vi "Day 4.vi"() -> ()   [LabVIEW 2020]
uses:
  Typedefs/Passport.ctl
  Typedefs/ecl.ctl
panel:
  out "Array 3":T1(array[cluster])
  out "Failures Only":string[](array[string])
  out "Array 2":bool[](array[boolean])
  out "sum":i16
  out "Array":T2[](array[typedef])
  out "output array":string[](array[string])
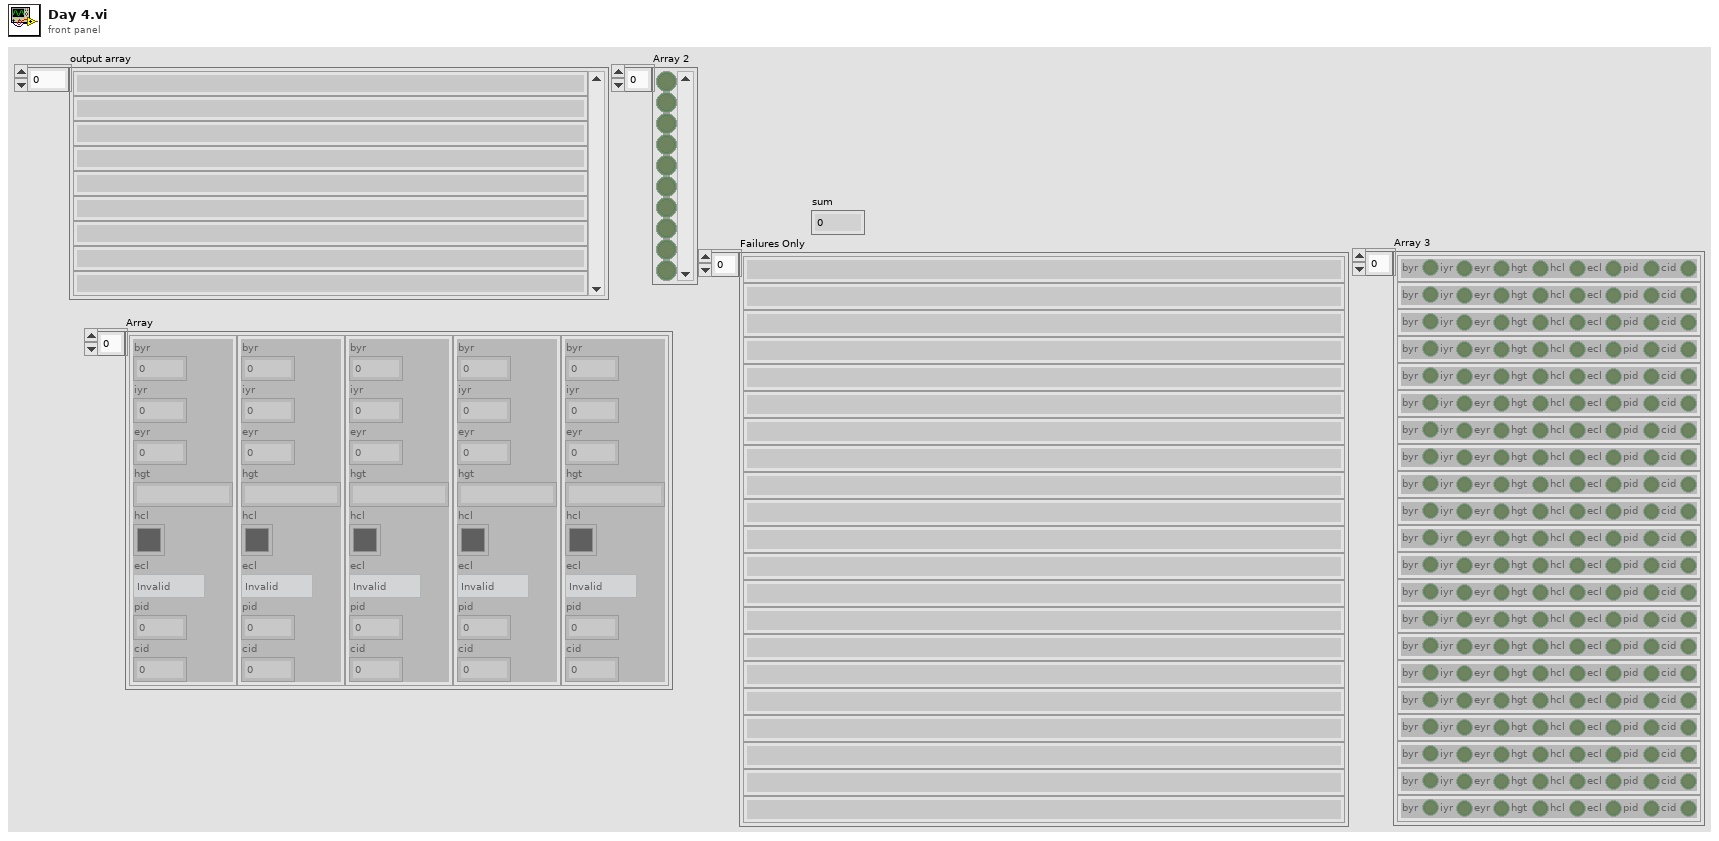
[diagram p1: front panel]
types:
  T1 = cluster{"byr":bool, "iyr":bool, "eyr":bool, "hgt":bool, "hcl":bool, "ecl":bool, "pid":bool, "cid":bool}[]
  T2 = typedef "Passport.ctl" = cluster{"byr":i32, "iyr":i32, "eyr":i32, "hgt":string, "hcl":u32, "ecl":T3, "pid":i32, "cid":i32}
  T3 = typedef "ecl.ctl" = enum16{"Invalid", "amb", "blu", "brn", "gry", "grn", "hzl", "oth"}
  T4 = cluster{"byr":bool, "iyr":bool, "eyr":bool, "hgt":bool, "hcl":bool, "ecl":bool, "pid":bool, "cid":bool}
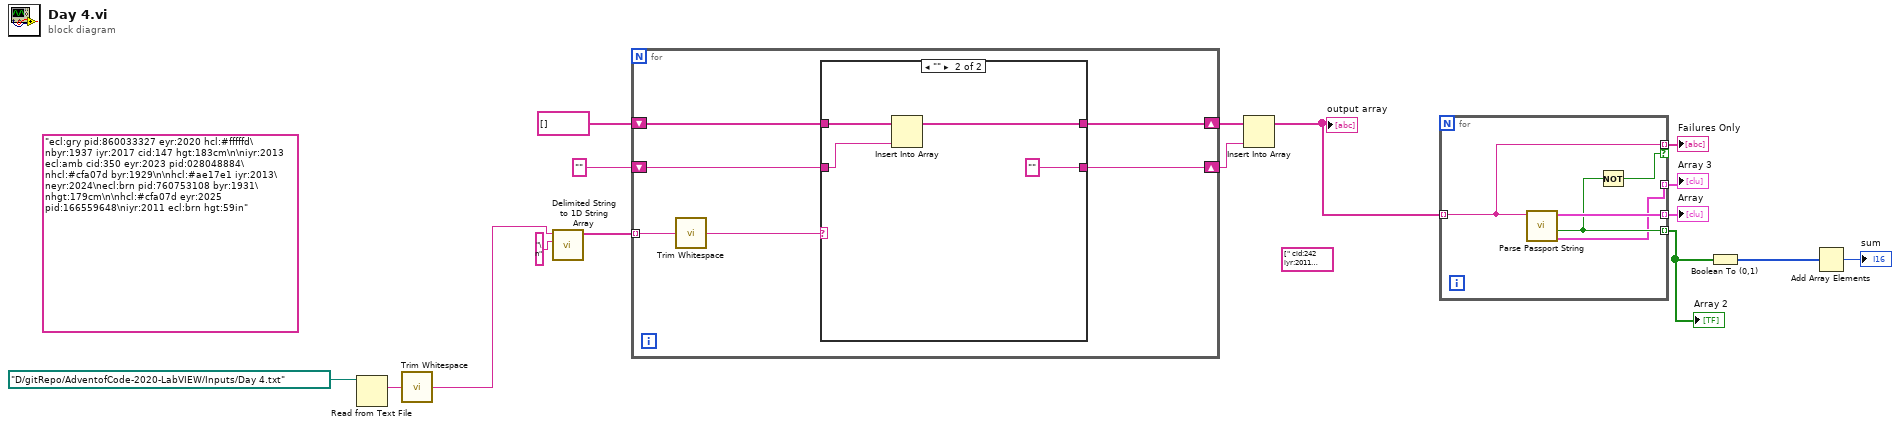
[diagram p0: block diagram]
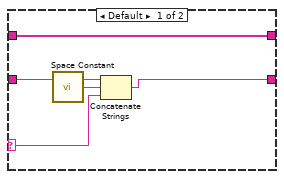
[diagram p2: hidden frame]
diagram:
  (unwired) string[] [" cid:242 iyr:2011 pid:953198122 eyr:2029 ecl:blu hcl:#888785", " hcl:#fffffd hgt:152cm byr:1996 ecl:gry eyr:2024", " pid:328737320 iyr:2017 hcl:#fffffd hgt:178 ecl:#35fad5 byr:1959", " iyr:2010 byr:1943 eyr:2028 hgt:178cm hcl:#888785 pid:572750267", " hgt:182cm ecl:blu eyr:2028 iyr:2011 hcl:#a97842 pid:758494126", " iyr:2023 hgt:174cm hcl:cafc2f ecl:utc cid:299 eyr:2026 pid:57963956", " ecl:amb hgt:70 iyr:2018 pid:241872490 byr:1962 eyr:2024 hcl:c5f0c3", " pid:994754974 eyr:2029 iyr:2017 cid:137 byr:1966 hcl:#733820 ecl:blu", " ecl:utc pid:937481632 hgt:190 eyr:2025 iyr:2027 byr:1949 cid:84 hcl:d3f4f5", " byr:2010 hgt:181cm iyr:2020 eyr:2040 pid:785862801 ecl:#f84ccd", " cid:314 hgt:180cm ecl:amb hcl:#602927 byr:2027 iyr:1958 eyr:2020 pid:#b2b732", " eyr:2030 pid:783631610 hgt:74 byr:2014 hcl:z iyr:2003 ecl:grt", " ecl:#d4d852 iyr:2029 hcl:z hgt:185in eyr:2034 pid:#526166", " iyr:1946 eyr:1957 byr:1941 pid:632690435 ecl:oth hcl:18a37c hgt:59cm", " iyr:2013 eyr:2026 pid:002380966 cid:95 hcl:#623a2f byr:1965 ecl:oth", " ecl:#5d8b3b hgt:156cm eyr:2029 pid:#3df0cc byr:1967 cid:118 hcl:e23f0f", " byr:1966 hgt:158cm eyr:2029 hcl:#602927 iyr:2013 pid:963663665", " hcl:#fffffd ecl:gry cid:93 pid:731904973 byr:1939 eyr:2029 iyr:2016", " pid:96716037 iyr:1938 eyr:2032 hgt:192 ecl:gmt byr:2029 hcl:02edc5", " byr:1958 iyr:2011 eyr:2029 ecl:gry pid:526931024 hcl:z hgt:59cm", " pid:1134356373 iyr:2019 ecl:grn hcl:#ceb3a1 byr:1950 hgt:154in", " hgt:157cm ecl:zzz byr:1976 pid:5047305958 iyr:2013 hcl:#341e13", " iyr:2029 ecl:#559ffe hcl:z cid:156 byr:2003 hgt:178 pid:93994500", " iyr:2026 hcl:#eda7f3 ecl:amb byr:1921 eyr:2021 pid:153cm", " pid:555636800 eyr:2020 hgt:182cm iyr:2019 byr:1948 cid:325 hcl:#733820", " eyr:1973 iyr:2024 hcl:z byr:2028 ecl:dne cid:169 pid:43596015 hgt:170in", " iyr:2013 hcl:z hgt:73cm byr:2014 pid:192cm ecl:#1627a7", " pid:816749378 hgt:178cm hcl:#733820 eyr:2029 byr:1993", " hcl:0cacc5 byr:1944 iyr:2028 eyr:2024 hgt:163in pid:74169361 ecl:dne", " hcl:#ceb3a1 ecl:grn eyr:2027 pid:481186415 hgt:176cm cid:325 byr:1986", " ecl:brn cid:323 hgt:167 byr:1993 iyr:1953 hcl:z eyr:2023 pid:161542750", " ecl:#895336 eyr:2033 hgt:67cm cid:254 iyr:1967 hcl:z byr:1954", " ecl:utc iyr:2014 hgt:183in byr:2007 eyr:2026 hcl:#cfa07d cid:334", " ecl:gry hcl:#b6652a pid:250420128 eyr:2024 byr:1939 hgt:170cm", " hgt:129 byr:2016 hcl:6734a1 ecl:#915282 iyr:1949 cid:130 pid:677408864 eyr:2030", " ecl:grn iyr:2019 pid:775867641 hcl:#bf1e29 byr:1920 hgt:163cm", " iyr:2019 ecl:#19fef5 pid:2080468234 eyr:2008 hgt:72 hcl:e14dfe byr:1980 cid:272", " byr:2025 cid:163 iyr:2020 pid:758946748 hgt:161cm ecl:amb eyr:2023 hcl:026d4d", " eyr:2023 hcl:z iyr:2019 byr:2013 ecl:#b42611 pid:164cm hgt:60cm", " cid:168 pid:#8556c9 hcl:413944 eyr:2036 byr:2013 iyr:2012 ecl:#66dc1c hgt:59cm", " eyr:1984 byr:2017 pid:#cbc84e hcl:z cid:189 iyr:2021 ecl:blu hgt:152cm", " hgt:172 byr:2008 eyr:2030 iyr:1959 ecl:oth hcl:#a8ebbb", " iyr:2013 hcl:#8f97b1 hgt:182cm ecl:grn cid:89 eyr:2029 byr:1974", " hcl:z pid:85905429 byr:1923 cid:260 eyr:2031 ecl:gry iyr:2022 hgt:180cm", " ecl:oth pid:087762106 hgt:190cm byr:1974 cid:171 hcl:#c63f21 eyr:2020", " hgt:170cm eyr:2021 cid:219 hcl:#a97842 pid:040224991 byr:1950 iyr:2018", " byr:2029 eyr:2036 cid:309 iyr:2016 hgt:167cm hcl:#fffffd ecl:#1ab23b", " eyr:2029 pid:669044398 hgt:161cm hcl:#cfa07d ecl:gry iyr:2018", " iyr:2013 eyr:2027 cid:223 pid:145547438 hcl:#6e6f47 hgt:165cm ecl:amb", " eyr:2026 hcl:z byr:2018 pid:7809314464 iyr:2012 hgt:158cm ecl:hzl", " cid:291 hgt:168 ecl:#7734de iyr:2021 hcl:5b4ef1 pid:3381158334 eyr:1956 byr:2003", " pid:68300657 byr:1988 hgt:181cm ecl:hzl iyr:1951 hcl:e18469 eyr:2013", " pid:157572693 hgt:185cm hcl:#065fe8 ecl:gry eyr:2027 iyr:2014", " eyr:2029 hgt:164cm hcl:z ecl:grn cid:270 iyr:2019 byr:1993 pid:338068138", " iyr:2019 eyr:2024 hgt:174cm pid:855792798 byr:1920 hcl:#cfa07d", " eyr:2020 hgt:74in iyr:2013 ecl:amb byr:1920 hcl:3f6214 pid:957164804", " byr:2021 hcl:ca4bcf hgt:88 iyr:2017 ecl:gmt pid:181cm eyr:2032", " iyr:2002 cid:139 byr:1982 hcl:#c0946f pid:#62721b hgt:159in eyr:1966 ecl:brn", " eyr:2036 ecl:oth byr:2026 hgt:96 pid:137651094 hcl:z", " pid:373485985 iyr:2030 ecl:gry byr:2011 hgt:65cm hcl:#733820", " pid:#fd3377 ecl:#618bce hcl:#ceb3a1 iyr:1944 hgt:182cm cid:57 byr:2022 eyr:1995", " pid:4790730010 hgt:192cm cid:222 byr:2022 hcl:4798e7 ecl:#5126d5 iyr:1954 eyr:2040", " iyr:1979 hcl:e09b9c byr:2016 hgt:121 eyr:1962 pid:#fb14be cid:265 ecl:lzr", " ecl:#fe1b74 iyr:1926 hgt:70cm pid:70807766 hcl:556dca byr:2030 eyr:2032", " eyr:2039 byr:2025 pid:247367429 hcl:z iyr:2013 ecl:amb cid:118", " eyr:2027 hcl:z ecl:utc cid:274 hgt:175in iyr:2016 byr:1977 pid:478855994", " ecl:utc byr:2026 iyr:1999 eyr:1937 hgt:66cm hcl:z pid:2247643960", " ecl:xry pid:346719476 iyr:1999 eyr:2020 hgt:154cm hcl:z byr:2027", " iyr:2010 hcl:#efcc98 pid:351846405 eyr:2024 hgt:150cm byr:1941", " byr:1994 eyr:2028 ecl:gry hcl:#888785 iyr:2010 hgt:165cm cid:183", " eyr:2031 hcl:6804ef ecl:amb byr:2024 hgt:157cm iyr:1938 pid:#0418fb", " pid:381452527 eyr:2027 hcl:#efcc98 ecl:brn byr:1956 hgt:63in", " byr:1968 pid:875469219 hcl:#efcc98 hgt:176cm cid:141 iyr:2017", " byr:1947 hcl:z cid:188 eyr:2038 pid:177cm iyr:2011 hgt:166cm ecl:#c1376b", " ecl:hzl hgt:170cm cid:307 eyr:2022 byr:1971 hcl:#b6652a pid:047040501", " hgt:126 ecl:zzz byr:2019 pid:170207910 eyr:2035 hcl:23df48 iyr:1932", " hgt:152cm cid:270 eyr:2036 ecl:#408f6e iyr:1952 pid:5808880830 byr:2022 hcl:0b1ba6", " hgt:67cm eyr:2028 pid:816355657 iyr:2019 byr:2008 hcl:z ecl:#5b4f31", " byr:1955 hgt:71in iyr:2018 pid:320019385 hcl:#6b5442 cid:324 eyr:2027", " pid:957860464 hcl:#602927 iyr:2011 byr:2026 cid:261 eyr:2006", " pid:#1742ae ecl:#a61090 iyr:2028 hcl:717dd0 hgt:139 cid:183 eyr:2035", " ecl:#4004e3 cid:278 iyr:1950 pid:745107377 byr:2007 eyr:2036 hcl:8447eb hgt:74cm", " hgt:187cm iyr:1921 ecl:#1c7d96 eyr:1987 byr:2028 pid:#28e5a1 cid:144 hcl:9fc25d", " pid:860410143 ecl:dne eyr:2031 cid:206 hgt:187in byr:1927 hcl:8c2149 iyr:2012", " iyr:2010 byr:1963 cid:139 pid:160019759 eyr:2030 hgt:172cm hcl:#602927", " byr:2023 ecl:brn cid:101 eyr:2016 pid:190078757 hgt:188in", " byr:2011 hcl:z ecl:gry pid:408316491 hgt:64cm iyr:2017 eyr:1968", " ecl:oth hcl:#6b5442 pid:623099801 hgt:163cm byr:1928", " pid:165230004 ecl:grn byr:1935 hcl:#c0946f iyr:2012 hgt:185cm", " ecl:#f3d8ba hgt:182cm eyr:2020 byr:2007 hcl:z iyr:2014 pid:6141297559", " pid:867747198 hcl:#efcc98 eyr:2030 byr:1989 hgt:181cm", " eyr:2034 hcl:#623a2f byr:1958 pid:60553207 ecl:#76b538 hgt:59 cid:75", " ecl:grn eyr:2036 iyr:1951 byr:2029 hcl:z hgt:177in pid:135470038", " byr:2014 pid:25253929 hcl:z ecl:#f3fb41 eyr:2025 cid:255 iyr:1998 hgt:155cm", " ecl:gry pid:919070381 hcl:#efcc98 iyr:2019 eyr:2021 byr:1995", " ecl:gry byr:1963 iyr:2016 hgt:188cm pid:024539026 eyr:2022", " iyr:2011 hcl:#888785 eyr:2030 ecl:gry byr:1920", " pid:#0468a7 hcl:851fe0 eyr:2036 hgt:60cm byr:2030 iyr:1995 ecl:utc", " cid:185 ecl:#5f6f53 pid:#20f317 byr:2024 eyr:1988 hcl:z iyr:2023 hgt:158in", " pid:782547454 hcl:z ecl:#b0805f iyr:2013 eyr:2023 hgt:159cm byr:1935 cid:230", " pid:298008321 hcl:231e1b hgt:166cm ecl:oth iyr:2026 eyr:2020", " pid:230201309 iyr:2010 eyr:2025 hcl:#6b5442 cid:238 ecl:grn hgt:174cm", " iyr:2020 byr:1938 pid:927067439 eyr:2027 hgt:173cm hcl:306963 ecl:xry", " byr:1991 iyr:2021 hgt:175cm hcl:68b4f3 ecl:utc pid:037777327 eyr:2026", " byr:1938 eyr:2021 pid:575395401 cid:234 hcl:#866857 ecl:hzl hgt:176cm", " hcl:#ceb3a1 ecl:hzl eyr:2035 iyr:2014 byr:2019", " eyr:1936 ecl:blu hgt:153cm hcl:98d3f0 pid:7296832671 byr:1931 iyr:1962", " pid:203025149 eyr:2029 iyr:2010 cid:124 byr:1999 ecl:blu", " iyr:2011 eyr:2028 pid:#7e0612 byr:1924 hcl:#7d3b0c ecl:oth hgt:82", " pid:#49ea2c eyr:2029 hcl:#6b5442 iyr:1931 hgt:62cm ecl:brn byr:2012", " eyr:2038 hcl:8d1f49 ecl:#6d4ea1 pid:0853660207 byr:2020 hgt:71cm", " byr:1921 hcl:#c0946f ecl:blu iyr:2019 eyr:2024 pid:643387204", " byr:2004 iyr:2022 pid:157cm eyr:2035 ecl:#eafe47 hgt:129 hcl:z", " byr:1930 hcl:5bdf31 pid:#b21f8a hgt:164cm cid:134 iyr:2023 ecl:lzr", " hcl:2a1c4f iyr:2011 hgt:192cm eyr:2028 byr:2029 cid:270 ecl:dne pid:7995627426", " eyr:2022 iyr:2018 byr:1972 cid:290 hgt:170cm ecl:grn pid:127269636", " pid:571765355 byr:2021 hcl:z eyr:1921 cid:106 iyr:1978 ecl:#1162c5 hgt:184in", " ecl:hzl pid:484466493 hgt:176cm iyr:2016 byr:1983 hcl:#ceb3a1", " ecl:brn hcl:352cf1 cid:149 hgt:184cm byr:2011 eyr:2031 pid:21942403 iyr:2028", " ecl:gry hcl:#18171d iyr:2015 hgt:185cm eyr:2023 byr:1950", " iyr:2003 eyr:2020 cid:99 byr:2027 hcl:2c10a6 hgt:74cm ecl:brn", " pid:151cm hcl:46a5fd eyr:2031 iyr:2014 byr:2005 ecl:xry hgt:176cm", " byr:2011 ecl:oth pid:821123244 iyr:2022 hcl:839b47 eyr:2039 hgt:150in", " iyr:2018 hgt:164cm hcl:#650d28 byr:1973 cid:108 pid:#b0df80 ecl:blu eyr:2020", " hcl:z pid:315901778 iyr:2013 byr:1999 ecl:#49f691 eyr:2026 hgt:179cm", " pid:163cm hgt:189cm iyr:1997 hcl:03db25 eyr:1970 byr:2016 ecl:#6c59eb", " pid:766719295 iyr:2017 hgt:168cm hcl:z ecl:grt eyr:2022 byr:2010", " hgt:173cm pid:247156751 cid:109 eyr:2022 iyr:2012 ecl:gry byr:1989", " cid:288 hcl:77241f hgt:157cm byr:1956 pid:587115461 iyr:2016 ecl:lzr eyr:2034", " hcl:5307c9 ecl:#cc4aff pid:#d80d30 cid:224 hgt:72cm byr:2025 eyr:2039 iyr:2025", " eyr:2027 byr:2015 hgt:184 hcl:98fb9d pid:58151347 iyr:2029"] ("Failures Only")
  (unwired) "ecl:gry pid:860033327 eyr:2020 hcl:#fffffd\nbyr:1937 iyr:2017 cid:147 hgt:183cm\n\niyr:2013 ecl:amb cid:350 eyr:2023 pid:028048884\nhcl:#cfa07d byr:1929\n\nhcl:#ae17e1 iyr:2013\neyr:2024\necl:brn pid:760753108 byr:1931\nhgt:179cm\n\nhcl:#cfa07d eyr:2025 pid:166559648\niyr:2011 ecl:brn hgt:59in"
  n1 = Read from Text File(file (use dialog)=path "D:/gitRepo/AdventofCode-2020-LabVIEW/Inputs/Day 4.txt" ("Path")) -> (text=w5:string)  [unwired: 3 in, 3 out]
  n2 = call <vilib>:"Trim Whitespace.vi"("string"=w5) -> ("trimmed string"=w4:string)  [unwired: 1 in]
  n3 = call <vilib>:"Delimited String to 1D String Array.vi"("delimiter"="\n", "delimited string"=w4) -> ("string array"=w15:string[])  [unwired: 9 in]
  n4 = for {
    tunnel: w15 -> [w22] mode=indexing
    shift-right: [w18] -> w12
    shift-left: string[] [] -> [w19]
    shift-right: [w20] -> w11
    shift-left: "" ("String") -> [w21]
    n5 = call <vilib>:"Trim Whitespace.vi"("string"=w22) -> ("trimmed string"=w17:string)  [unwired: 1 in]
    n6 = case shown="\"\"" w17 {
      selector: w17 -> [w24 _]
      tunnel: w21 -> [w26 w29]
      tunnel: [w25 "" ("String")] -> w20
      tunnel: w19 -> [w27 w30]
      tunnel: [w27 w28] -> w18
      frame Default {
        n7 = call <vilib>:"Space Constant.vi"() -> ("String"=w23:string)
        n8 = Concatenate Strings(w26, w23, w24) -> (w25:string)
      }
      frame "" {
        n9 = Insert Into Array(array=w30, new element=w29) -> (w28:string[])  [unwired: 1 in]
      }
    }
  }
  n10 = Insert Into Array(array=w12, new element=w11) -> (w2:string[])  [unwired: 1 in]
  "output array" <- w2
  n11 = for {
    tunnel: w2 -> [w35] mode=indexing
    tunnel: [w36] -> w10 mode=indexing
    tunnel: [w34] -> w9 mode=indexing
    tunnel: [w35] -> w3 mode=indexing if=w33
    tunnel: [w32] -> w1 mode=indexing
    n12 = call "Parse Passport String.vi"("Passport String"=w35) -> ("Why Bad"=w32:T4, "Valid?"=w34:bool, "Passport Info"=w36:T2)  [unwired: 8 in]
    n13 = Not(x=w34) -> (.not. x?=w33:bool)
  }
  "Array" <- w10
  "Array 2" <- w9
  "Failures Only" <- w3
  "Array 3" <- w1
  n14 = Boolean To (0,1)(Boolean=w9) -> (0, 1=w8:i16[])
  n15 = Add Array Elements(numeric array=w8) -> (sum=→"sum":i16)
